vi "CSM Data Type String to Enum(String).vi"(10 "Data Type String":string) -> (1 "Array Dim":i32, 2 "Secondary Type String":string, 3 "Primary Type":T1)   [LabVIEW 2020, in "Communicable State Machine.lvlib"]
uses:
  Communicable State Machine.lvlib
  Data Type.ctl
  Refnum Type.ctl
  NI_Data Type.lvlib
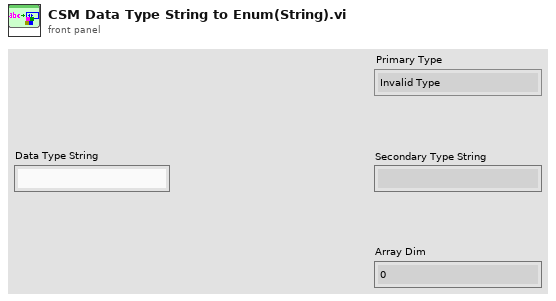
[diagram p1: front panel]
types:
  T1 = typedef "NI_Data Type.lvlib/Data Type.ctl" = enum8{"Invalid Type", "Void", "I8", "I16", "I32", "I64", "U8", "U16", "U32", "U64", "Single Float", "Double Float", "Extended Float", "Single Complex", "Double Complex", "Extended Complex", "Enum U8", "Enum U16", "Enum U32", "Enum U64", "Single Float With Unit", "Double Float With Unit", "Extended Float With Unit", "Single Complex with Unit", "Double Complex with Unit", "Extended Complex with Unit", "Boolean", "String", "Path", "Picture", "Tag", "Array", "Cluster", "Variant", "LV Variant", "Waveform", "Timestamp", "Digital Waveform", "Digital Data", "ExpressData", "Refnum", "External Data", "VI", "Poly VI", "LabVIEW Class Instance", "Fixed Point", "Set Collection", "Map Collection"}
  T2 = typedef "NI_Data Type.lvlib/Refnum Type.ctl" = enum16{"NotARefnum", "UnknownRefnum", "Generic", "Datalog", "ByteStream", "Device", "Occurence", "TCPNetConnection", "Auto", "Menu", "Imaq", "Hardware", "DataSocket", "Visa", "IVI", "UDPNetConnection", "Notifier", "Queue", "Irda", "EventReg", "DotNet", "UserEvent", "Callback", "UNUSED_EMPTY_POSITION", "BlueToothNetConnection", "LVObjApp", "LVObjVI", "LVObjUnknown", "GenericClass", "UserDefinedRefnumTag", "DataValue", "RT FIFO", "TDMS File", "PythonSessionRefnum"}
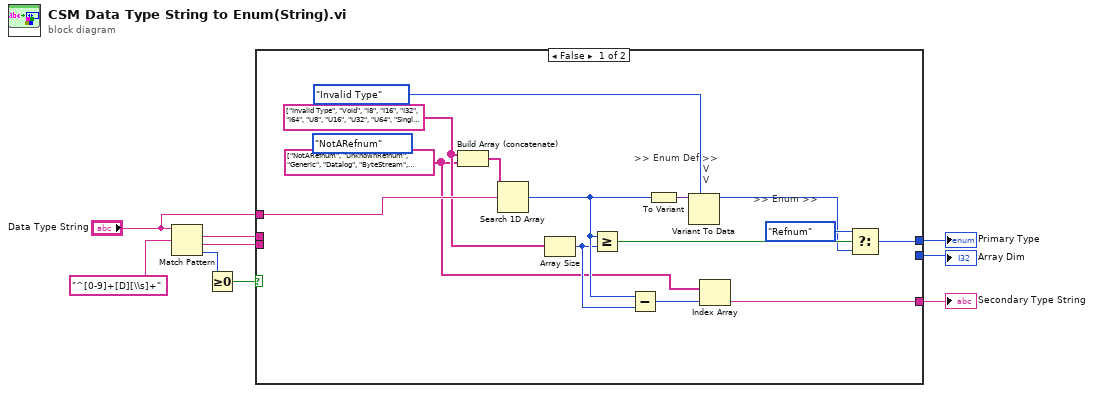
[diagram p0: block diagram]
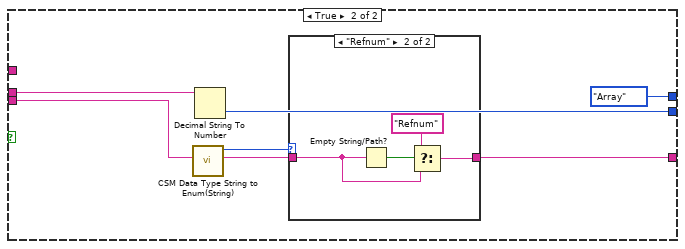
[diagram p2: hidden frame]
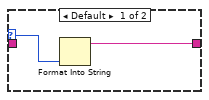
[diagram p3: hidden frame]
diagram:
  n1 = Match Pattern(string="Data Type String", regular expression="^[0-9]+[D][\\s]+") -> (match substring=w7:string, after substring=w3:string, offset past match=w8:i32)  [unwired: 1 in, 1 out]
  n2 = Greater Or Equal To 0?(x=w8) -> (x >= 0?=w6:bool)
  n3 = case shown="False" w6 {
    tunnel: w7 -> [_ w30]
    tunnel: [w15 Data_Type."Array" ("Type")] -> w5
    tunnel: [_ w28] -> w4
    tunnel: w3 -> [_ w27]
    tunnel: [w10 w25] -> w2
    tunnel: "Data Type String" -> [w22 _]
    frame False {
      (unwired) Refnum_Type."NotARefnum" ("Reference Type")
      w11 = string[] ["NotARefnum", "UnknownRefnum", "Generic", "Datalog", "ByteStream", "Device", "Occurence", "TCPNetConnection", "Auto", "Menu", "Imaq", "Hardware", "DataSocket", "Visa", "IVI", "UDPNetConnection", "Notifier", "Queue", "Irda", "EventReg", "DotNet", "UserEvent", "Callback", "UNUSED_EMPTY_POSITION", "BlueToothNetConnection", "LVObjApp", "LVObjVI", "LVObjUnknown", "GenericClass", "UserDefinedRefnumTag", "DataValue", "RT FIFO", "TDMS File"] ("Enum Strings")
      w19 = string[] ["Invalid Type", "Void", "I8", "I16", "I32", "I64", "U8", "U16", "U32", "U64", "Single Float", "Double Float", "Extended Float", "Single Complex", "Double Complex", "Extended Complex", "Enum U8", "Enum U16", "Enum U32", "Enum U64", "Single Float With Unit", "Double Float With Unit", "Extended Float With Unit", "Single Complex with Unit", "Double Complex with Unit", "Extended Complex with Unit", "Boolean", "String", "Path", "Picture", "Tag", "Array", "Cluster", "Variant", "LV Variant", "Waveform", "Timestamp", "Digital Waveform", "Digital Data", "ExpressData", "Refnum", "External Data", "VI", "Poly VI", "LabVIEW Class Instance", "Fixed Point"] ("Enum Strings")
      # ">> Enum >>"
      # ">> Enum Def >>\n                       V\n                       V"
      n4 = Build Array (concatenate)(w19, w11) -> (w23:string[])
      n5 = Search 1D Array(1D array=w23, element=w22) -> (index of element=w14:i32)  [unwired: 1 in]
      n6 = Array Size(array=w19) -> (size(s)=w13:i32)
      n7 = Greater Or Equal?(x=w14, y=w13) -> (x >= y?=w18:bool)
      n8 = Subtract(x=w14, y=w13) -> (x-y=w12:i32)
      n9 = To Variant(anything=w14) -> (Variant=w21:variant)
      n10 = Variant To Data(type=Data_Type."Invalid Type" ("Type"), Variant=w21) -> (data=w16:T1)  [unwired: 1 in, 1 out]
      n11 = Index Array(array=w11, index=w12) -> (element=w10:string)
      n12 = Select(t=Data_Type."Refnum", s=w18, f=w16) -> (s? t:f=w15:T1)
    }
    frame True {
      n13 = call "CSM Data Type String to Enum(String).vi"("Data Type String"=w27) -> ("Secondary Type String"=w24:string, "Primary Type"=w26:T1)  [unwired: 8 in, 1 out]
      n14 = Decimal String To Number(string=w30) -> (number=w28:i32)  [unwired: 2 in, 1 out]
      n15 = case shown="\"Refnum\"" w26 {
        selector: w26 -> [w32 _]
        tunnel: [w31 w33] -> w25
        tunnel: w24 -> [_ w35]
        frame Default {
          n16 = Format Into String(w32) -> (resulting string=w31:string)  [unwired: 3 in, 1 out]
        }
        frame "Refnum" {
          n17 = Empty String/Path?(string/path=w35) -> (empty?=w36:bool)
          n18 = Select(t="Refnum", s=w36, f=w35) -> (s? t:f=w33:string)
        }
      }
    }
  }
  "Primary Type" <- w5
  "Array Dim" <- w4
  "Secondary Type String" <- w2
